vi "Pre-Build Action.vi"(6 "Top Level/Always Included VIs":path[](array[path]), 7 "Main Destination Path":path, 9 "Target Name":string, 10 "Build Specification Name":string, 11 "Project Path":path) -> (0 "error out":errorcluster)   [LabVIEW 2016]
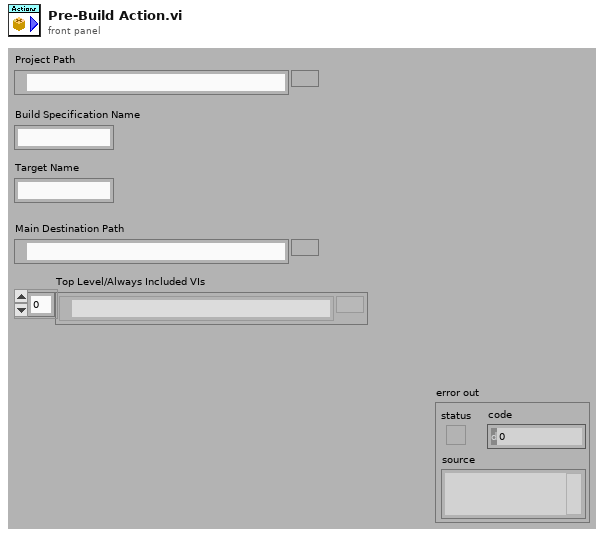
[diagram p1: front panel]
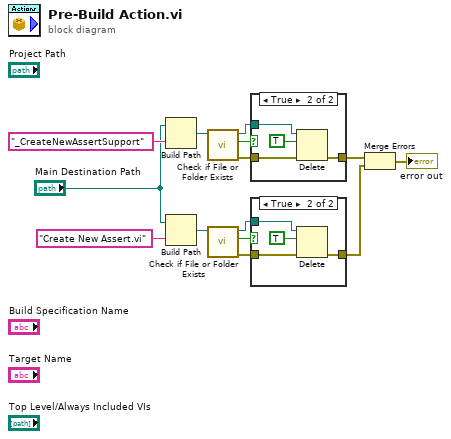
[diagram p0: block diagram]
diagram:
  n1 = Build Path(base path="Main Destination Path", name or relative path="_CreateNewAssertSupport") -> (appended path=w14:path)
  n2 = Build Path(base path="Main Destination Path", name or relative path="Create New Assert.vi") -> (appended path=w10:path)
  n3 = call <vilib>:"Check if File or Folder Exists.vi"("path"=w14) -> ("error out"=w7:errorcluster, "file or folder exists?"=w9:bool, "dup path"=w8:path)  [unwired: 8 in]
  n4 = call <vilib>:"Check if File or Folder Exists.vi"("path"=w10) -> ("error out"=w4:errorcluster, "file or folder exists?"=w6:bool, "dup path"=w5:path)  [unwired: 8 in]
  n5 = case shown="True" w9 {
    tunnel: w8 -> [_ w19]
    tunnel: w7 -> [w15 w17]
    tunnel: [w15 w16] -> w2
    frame False {
    }
    frame True {
      n6 = Delete(path (use dialog)=w19, entire hierarchy (F)=TRUE, error in=w17) -> (error out=w16:errorcluster)  [unwired: 2 in, 2 out]
    }
  }
  n7 = case shown="True" w6 {
    tunnel: w5 -> [_ w24]
    tunnel: w4 -> [w20 w22]
    tunnel: [w20 w21] -> w3
    frame False {
    }
    frame True {
      n8 = Delete(path (use dialog)=w24, entire hierarchy (F)=TRUE, error in=w22) -> (error out=w21:errorcluster)  [unwired: 2 in, 2 out]
    }
  }
  n9 = Merge Errors(w2, w3) -> (→"error out":errorcluster)
